vi "PH_ImageOperator.ProcEvents.vi"(0 "i ref in":refnum<vi>, 5 "error in (no error)":errorcluster) -> (14 "i ref out":refnum<vi>, 19 "error out":errorcluster)   [LabVIEW 2014, in "PH_ImageOperator.lvlib"]
doc: "This method is used to define the events the object will listen to. Add your own events here."
uses:
  PH_ImageOperator.lvlib
  CSCore/BaseProcess/BaseProcess.event definition.ctl
  CSCore/CAEObj/CAEObj.event definition.ctl
  CSCore/BaseProcess/BaseProcess.descriptor string definition.ctl
  CSCore/BaseProcess/BaseProcess.lvlib
  CSCore/CAEObj/CAEObj.lvlib
  PH_Common/PH_Common.lvlib
  PH_Img_BaseClass/PH_Img_BaseClass.lvlib
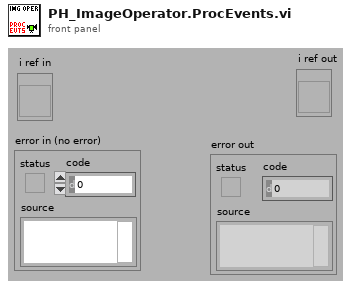
[diagram p1: front panel]
types:
  T1 = typedef "BaseProcess.lvlib/BaseProcess.event definition.ctl" = cluster{"CAEEvtDef":T2, "Data Descriptor":T3}
  T2 = typedef "CAEObj.lvlib/CAEObj.event definition.ctl" = cluster{"URL":string, "enable":bool, "ignoreResID":bool}
  T3 = typedef "BaseProcess.lvlib/BaseProcess.descriptor string definition.ctl" = string
  T4 = typedef "PH_Img_BaseClass.lvlib/PH_Img_BaseClass.i attribute.ctl" = cluster{"GUI Refs":T5, "Timeout Image [ms]":i32, "Default Periodic Period [ms]":i32, "Camera":cluster{"Instancename":string, "Notifier":refnum<notifier>}, "Palette":T6, "Cam Settings":cluster{"Cam ID":string, "Gain":dbl, "Brightness":dbl, "Shutter":dbl, "Cam Info Failure":bool, "Mode":i32}}
  T5 = typedef "PH_Img_BaseClass.lvlib/PH_Img_BaseClass.GUI Refs.ctl" = cluster{"Timeout":refnum<vi>, "Image":refnum<vi>, "Palette":refnum<vi>, "Timeout Set":refnum<vi>}
  T6 = typedef "PH_Img_BaseClass.lvlib/PH_Img_BaseClass.Palette.ctl" = i32
  T7 = typedef "PH_Common.lvlib/PH_DIM.Event Declarer.ctl" = cluster{"Service Name":string, "Selector":string}
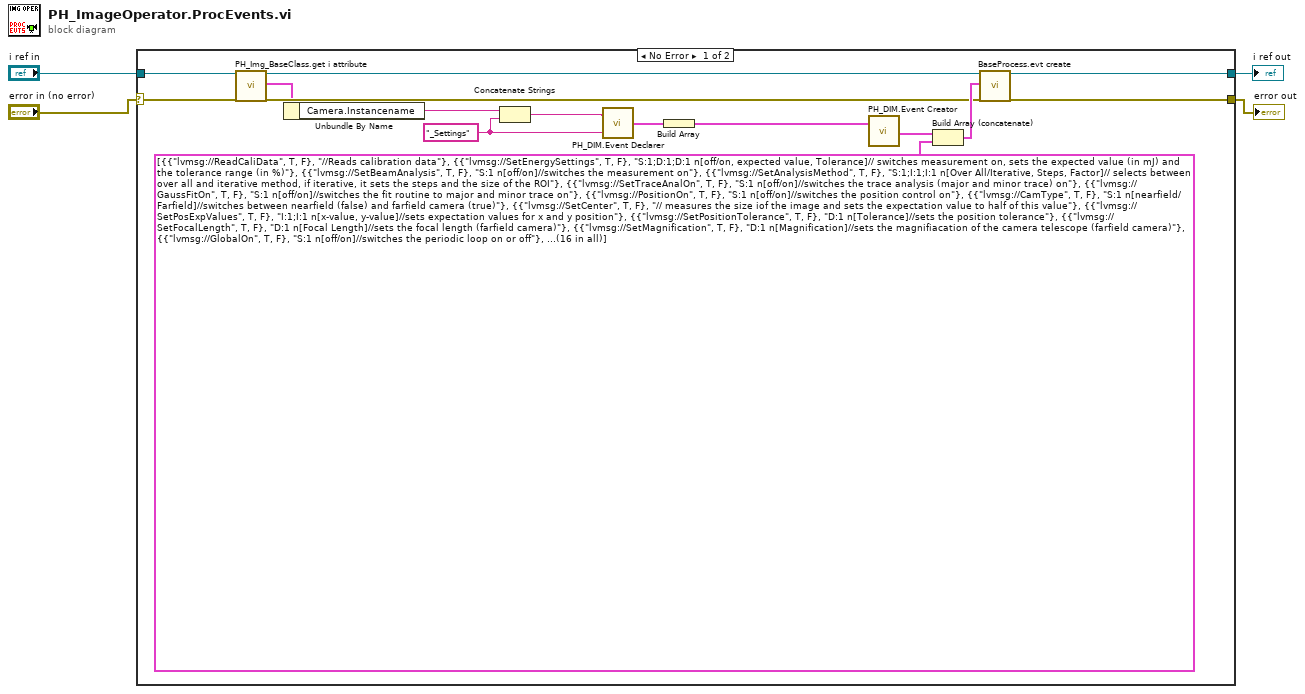
[diagram p0: block diagram]
diagram:
  n1 = case shown="No Error" "error in (no error)" {
    selector: "error in (no error)" -> [w11 w21]
    tunnel: "i ref in" -> [w13 w20]
    tunnel: [w19 w20] -> w3
    tunnel: [w18 w21] -> w2
    frame No Error {
      w6 = "_Settings" ("Service Name")
      n2 = call "PH_Img_BaseClass.get i attribute.vi"("i ref in"=w13, "error in (no error)"=w11) -> ("i ref out"=w12:refnum<vi>, "i attribute"=w9:T4, "error out"=w10:errorcluster)  [unwired: 15 in]
      n3 = Unbundle By Name(w9) -> ("Camera.Instancename"=w8:string)
      n4 = Concatenate Strings(w8, w6) -> (w5:string)
      n5 = call "PH_DIM.Event Declarer.vi"("Selector"=w6, "Service Name"=w5) -> ("declared DIM Event"=w7:T7)
      n6 = Build Array(w7) -> (w16:T7[])
      n7 = call "PH_DIM.Event Creator.vi"("Trendmessage Services"=w16) -> ("DIM Service Events"=w17:T1[])  [unwired: 18 in]
      n8 = Build Array (concatenate)(w17, T1[] [{"CAEEvtDef"={"URL"="lvmsg://ReadCaliData", "enable"=TRUE, "ignoreResID"=FALSE}, "Data Descriptor"="//Reads calibration data"}, {"CAEEvtDef"={"URL"="lvmsg://SetEnergySettings", "enable"=TRUE, "ignoreResID"=FALSE}, "Data Descriptor"="S:1;D:1;D:1 n[off/on, expected value, Tolerance]// switches measurement on, sets the expected value (in mJ) and the tolerance range (in %)"}, {"CAEEvtDef"={"URL"="lvmsg://SetBeamAnalysis", "enable"=TRUE, "ignoreResID"=FALSE}, "Data Descriptor"="S:1 n[off/on]//switches the measurement on"}, {"CAEEvtDef"={"URL"="lvmsg://SetAnalysisMethod", "enable"=TRUE, "ignoreResID"=FALSE}, "Data Descriptor"="S:1;I:1;I:1 n[Over All/Iterative, Steps, Factor]// selects between over all and iterative method, if iterative, it sets the steps and the size of the ROI"}, {"CAEEvtDef"={"URL"="lvmsg://SetTraceAnalOn", "enable"=TRUE, "ignoreResID"=FALSE}, "Data Descriptor"="S:1 n[off/on]//switches the trace analysis (major and minor trace) on"}, {"CAEEvtDef"={"URL"="lvmsg://GaussFitOn", "enable"=TRUE, "ignoreResID"=FALSE}, "Data Descriptor"="S:1 n[off/on]//switches the fit routine to major and minor trace on"}, {"CAEEvtDef"={"URL"="lvmsg://PositionOn", "enable"=TRUE, "ignoreResID"=FALSE}, "Data Descriptor"="S:1 n[off/on]//switches the position control on"}, {"CAEEvtDef"={"URL"="lvmsg://CamType", "enable"=TRUE, "ignoreResID"=FALSE}, "Data Descriptor"="S:1 n[nearfield/Farfield]//switches between nearfield (false) and farfield camera (true)"}, {"CAEEvtDef"={"URL"="lvmsg://SetCenter", "enable"=TRUE, "ignoreResID"=FALSE}, "Data Descriptor"="// measures the size iof the image and sets the expectation value to half of this value"}, {"CAEEvtDef"={"URL"="lvmsg://SetPosExpValues", "enable"=TRUE, "ignoreResID"=FALSE}, "Data Descriptor"="I:1;I:1 n[x-value, y-value]//sets expectation values for x and y position"}, {"CAEEvtDef"={"URL"="lvmsg://SetPositionTolerance", "enable"=TRUE, "ignoreResID"=FALSE}, "Data Descriptor"="D:1 n[Tolerance]//sets the position tolerance"}, {"CAEEvtDef"={"URL"="lvmsg://SetFocalLength", "enable"=TRUE, "ignoreResID"=FALSE}, "Data Descriptor"="D:1 n[Focal Length]//sets the focal length (farfield camera)"}, {"CAEEvtDef"={"URL"="lvmsg://SetMagnification", "enable"=TRUE, "ignoreResID"=FALSE}, "Data Descriptor"="D:1 n[Magnification]//sets the magnifiacation of the camera telescope (farfield camera)"}, {"CAEEvtDef"={"URL"="lvmsg://GlobalOn", "enable"=TRUE, "ignoreResID"=FALSE}, "Data Descriptor"="S:1 n[off/on]//switches the periodic loop on or off"}, {"CAEEvtDef"={"URL"="lvmsg://NoOffset", "enable"=TRUE, "ignoreResID"=FALSE}, "Data Descriptor"="S:1 n[off/on]//selects between Gaussian fit function with or without offset"}, {"CAEEvtDef"={"URL"="lvmsg://SetFFSettings", "enable"=TRUE, "ignoreResID"=FALSE}, "Data Descriptor"="S:1;S:1;D:1;D:1 n[off/on, Filter, Threshold, Damage Threshold]//Sets the Fill Factor Measurement; Damage Threshold is set in J/cm² "}] ("new events(V3.0)")) -> (w15:T1[])
      n9 = call "BaseProcess.evt create.vi"("i ref in"=w12, "newEvents"=w15, "error in (no error)"=w10) -> ("i ref out"=w19:refnum<vi>, "error out"=w18:errorcluster)  [unwired: 13 in, 2 out]
    }
    frame Error {
    }
  }
  "i ref out" <- w3
  "error out" <- w2
